vi "Write Config.vi"(8 "error in (no error)":errorcluster, 9 "Re-Init?":bool, 10 "ICM File In":path, 11 "Polynomial in":refnum<class "Polynomial.lvclass">) -> (0 "error out":errorcluster, 3 "Polynomial out":refnum<class "Polynomial.lvclass">)   [LabVIEW 2024, in "Polynomial.lvclass"]
doc: "Polynomial.lvclass:Write Config.vi\n\nThis VI writes the Polynomial Class parameters to the ICM configuration file.\n\nInstrument Communication Module Version 1.0\nSeptember, 2017 Original Code Consulting David Thomson\n www.originalcode.com"
uses:
  Polynomial.lvclass
  Polynomial.lvclass/Polynomial.ctl
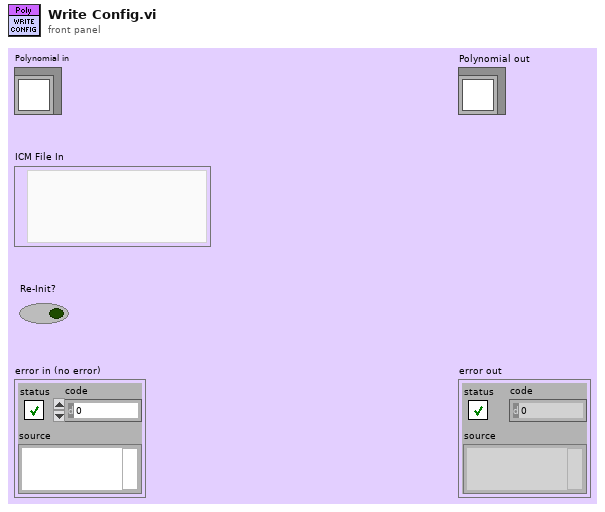
[diagram p1: front panel]
types:
  T1 = typedef "Polynomial Config.ctl" = cluster{"Polynomials":cluster{"Instance":string, "Polynomial":dbl[]}[]}
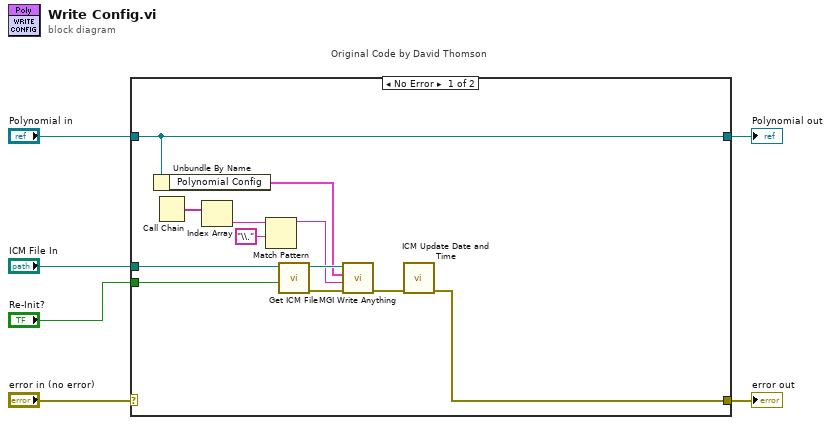
[diagram p0: block diagram]
diagram:
  n1 = case "Original Code by David Thomson" shown="No Error" "error in (no error)" {
    selector: "error in (no error)" -> [_ w20]
    tunnel: [w7 w20] -> w5
    tunnel: [w18 w19] -> w3
    tunnel: "Polynomial in" -> [w18 w19]
    tunnel: "ICM File In" -> [w14 _]
    tunnel: "Re-Init?" -> [w13 _]
    frame No Error {
      n2 = Unbundle By Name(w18) -> ("Polynomial Config"=w15:T1)
      n3 = Call Chain() -> (call chain=w11:string[])
      n4 = Index Array(array=w11) -> (element=w10:string)  [unwired: 1 in]
      n5 = Match Pattern(string=w10, regular expression="\\.") -> (before substring=w9:string)  [unwired: 1 in, 3 out]
      n6 = call "Get ICM File.vi"("Re-Init?"=w13, "ICM File In"=w14) -> ("error out"=w17:errorcluster, "ICM File"=w16:path)  [unwired: 8 in]
      n7 = call "MGI Write Anything.vi"("Error In"=w17, "Section Name (Name of \"Anything\")"=w9, "Anything"=w15, "Path (dialog)"=w16) -> ("Error Out"=w8:errorcluster)  [unwired: 5 in, 2 out]
      n8 = call "ICM Update Date and Time.vi"("error in (no error)"=w8) -> ("error out"=w7:errorcluster)  [unwired: 9 in, 1 out]
    }
    frame Error {
    }
  }
  "error out" <- w5
  "Polynomial out" <- w3
